vi "Read Elements.vi"(8 "error in (no error)":errorcluster, 11 "HC-ScanParser in":refnum<class "MC-ScanParser.lvclass">) -> (0 "error out":errorcluster, 2 "Elements":refnum<class "Element-XML.lvclass">[](array[class]), 3 "HC-ScanParser out":refnum<class "MC-ScanParser.lvclass">)   [LabVIEW 2013, in "MaterialCharacterization.lvlib" / "MC-ScanParser.lvclass"]
uses:
  MC-ScanParser.lvclass
  SM1000-XML/Element-XML/Element-XML.lvclass
  MC-ScanParser.lvclass/MC-ScanParser.ctl
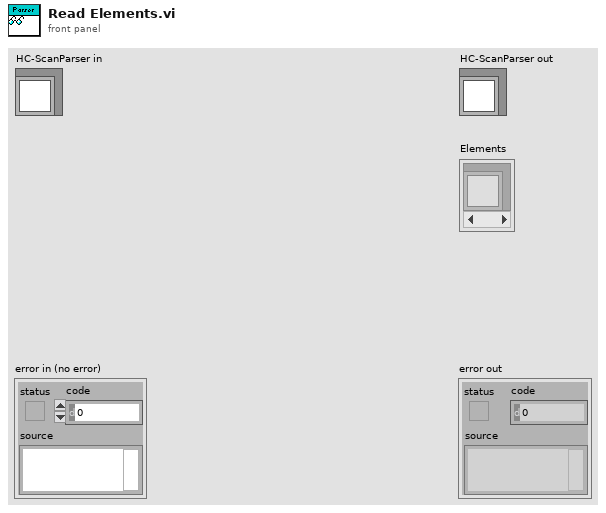
[diagram p1: front panel]
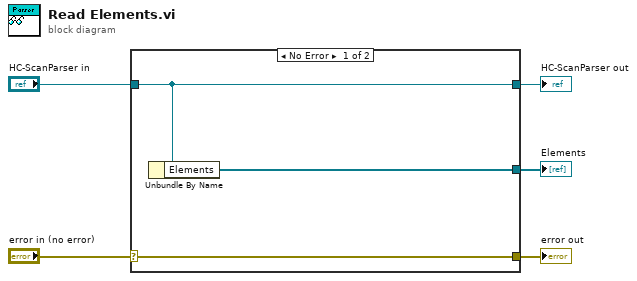
[diagram p0: block diagram]
diagram:
  n1 = case shown="No Error" "error in (no error)" {
    selector: "error in (no error)" -> [w8 w9]
    tunnel: [w8 w9] -> w4
    tunnel: [w7 w10] -> w2
    tunnel: "HC-ScanParser in" -> [w7 w10]
    tunnel: [w6 _] -> w1
    frame No Error {
      n2 = Unbundle By Name(w7) -> ("Elements"=w6:refnum<class "Element-XML.lvclass">[])
    }
    frame Error {
    }
  }
  "error out" <- w4
  "HC-ScanParser out" <- w2
  "Elements" <- w1
